vi "DOCustomPatternBuildArray.vi"(0 "object in":refnum<class "AD2_DO_SDK.lvclass">, 2 "Data":bool[](array[boolean]), 5 "error in (no error)":errorcluster) -> (14 "object out":refnum<class "AD2_DO_SDK.lvclass">, 16 "Array":u8[](array[numeric]), 19 "error out":errorcluster)   [LabVIEW 2021, in "AD2_DO_SDK.lvclass"]
uses:
  AD2_DO_SDK.lvclass
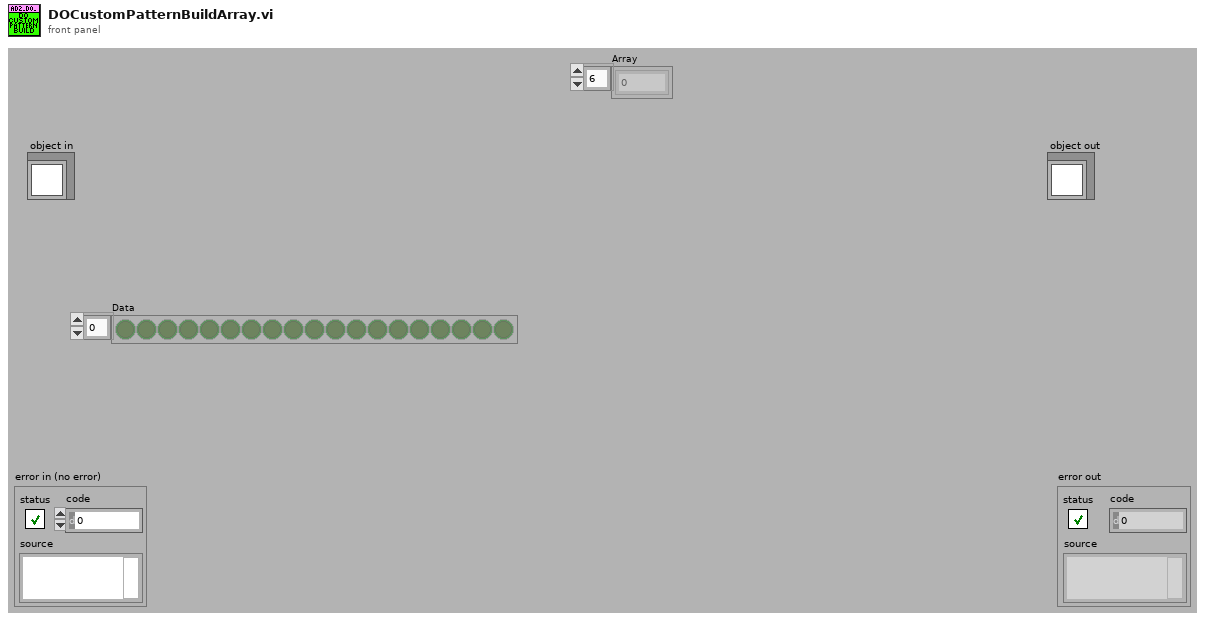
[diagram p1: front panel]
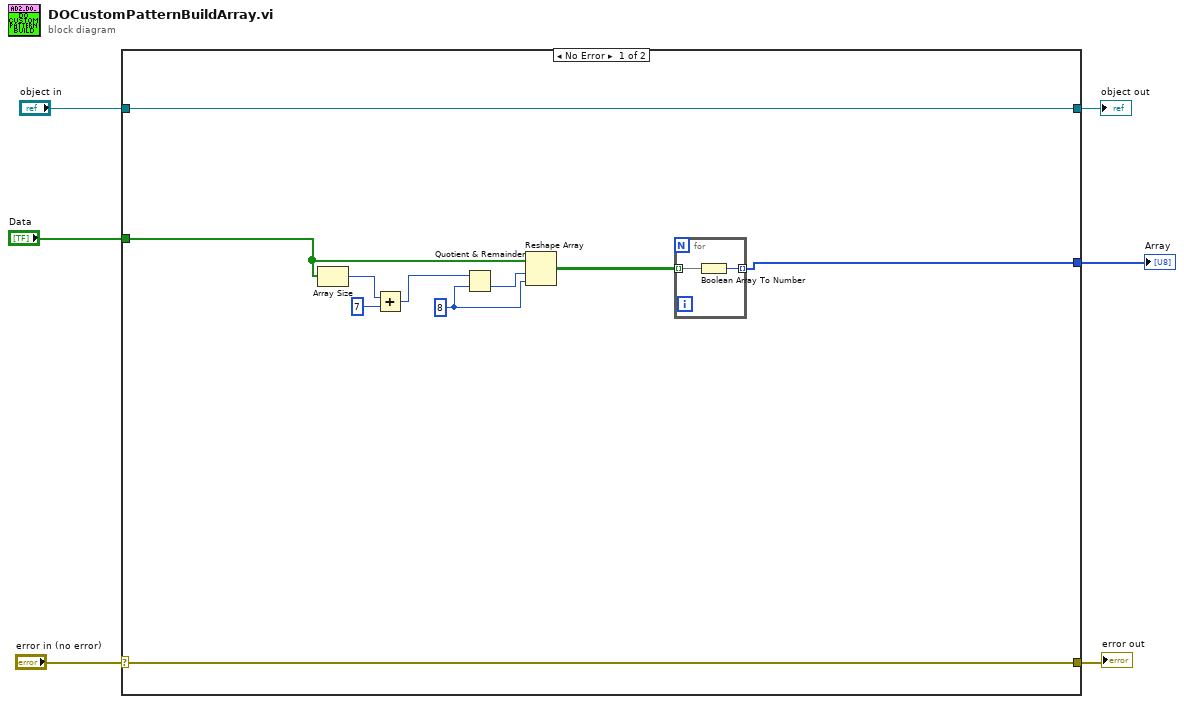
[diagram p0: block diagram]
diagram:
  n1 = case shown="No Error" "error in (no error)" {
    selector: "error in (no error)" -> [w16 w20]
    tunnel: [w16 w20] -> w5
    tunnel: [w15 w19] -> w3
    tunnel: "object in" -> [w15 w19]
    tunnel: "Data" -> [w10 _]
    tunnel: [w11 _] -> w1
    frame No Error {
      w14 = 8 ("y")
      n2 = Array Size(array=w10) -> (size(s)=w9:i32)
      n3 = Add(x=w9, y=7) -> (x+y=w8:i32)
      n4 = Quotient & Remainder(x=w8, y=w14) -> (floor(x/y)=w13:i32)  [unwired: 1 out]
      n5 = Reshape Array(w10, w13, w14) -> (w12:bool[][])
      n6 = for {
        tunnel: [w18] -> w11 mode=indexing
        tunnel: w12 -> [w17] mode=indexing
        n7 = Boolean Array To Number(Boolean array=w17) -> (number=w18:u8)
      }
    }
    frame Error {
    }
  }
  "error out" <- w5
  "object out" <- w3
  "Array" <- w1
